vi "To XML.vi"(8 "error in (no error)":errorcluster, 11 "Topic in":refnum<class "Topic.lvclass">) -> (0 "error out":errorcluster, 2 "XML String":string, 3 "Topic out":refnum<class "Topic.lvclass">)   [LabVIEW 2027, in "Topic.lvclass"]
uses:
  Topic.lvclass
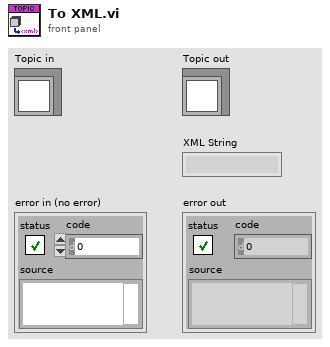
[diagram p1: front panel]
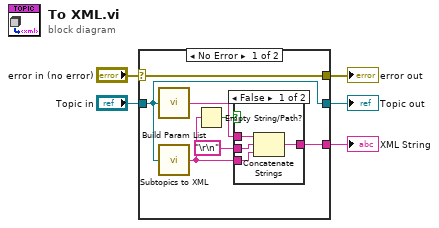
[diagram p0: block diagram]
diagram:
  n1 = case shown="No Error" "error in (no error)" {
    selector: "error in (no error)" -> [w12 w19]
    tunnel: [w12 w19] -> w4
    tunnel: [w6 w18] -> w2
    tunnel: "Topic in" -> [w6 w18]
    tunnel: [w10 _] -> w1
    frame No Error {
      n2 = call "Build Param List.vi"("Topic.lvclass"=w6) -> ("tagged string"=w11:string)
      n3 = call "Subtopics to XML.vi"("Topic in"=w6) -> ("tagged string"=w8:string)
      n4 = Empty String/Path?(string/path=w8) -> (empty?=w7:bool)
      n5 = case shown="False" w7 {
        tunnel: w11 -> [w16 w17]
        tunnel: [w15 w17] -> w10
        tunnel: "\r\n" -> [w14 _]
        tunnel: w8 -> [w13 _]
        frame False {
          n6 = Concatenate Strings(w16, w14, w13) -> (w15:string)
        }
        frame True {
        }
      }
    }
    frame Error {
    }
  }
  "error out" <- w4
  "Topic out" <- w2
  "XML String" <- w1
